vi "LoadCellTest.vi"() -> ()   [LabVIEW 2016]
uses:
  ModbusFactory/ModbusFactory.lvclass
  Common_RT_HPILC/HPILCFactory/HPILCFactory.lvclass
  Common_RT_HPILC/DataTypes/HPSettings.ctl
  Common_RT_ILC/DataTypes/ILCSettings.ctl
  Common_RT_ILC/DataTypes/ILCTimings.ctl
  Common_RT_HPILC/DataTypes/HPTimings.ctl
  ModbusFactory/ModbusFactory.lvclass/ModbusFactory.ctl
  Common_RT_ILC/ILC/ILC.lvclass/ILC.ctl
  <vilib>/Platform/TimedLoop/XDataNode/timing_clust.ctl
  <vilib>/Platform/TimedLoop/XDataNode/nitl_modes.ctl
  <vilib>/Platform/TimedLoop/XDataNode/wakeup.ctl
  Common_RT_Modbus/DynamicFrameParser/DynamicFrameParser.lvclass
  Common_RT_HPILC/HPILC/HPILC.lvclass/HPILC.ctl
  Common_RT_HPILC/HPILC/HPILC.lvclass
  D:/Code/Common_RT_ILC/ILC/ILC.lvclass
  <vilib>/FPGAPlugInAG/cRIO-9038/niLvFpga_Open_cRIO-9038.vi
  <vilib>/rvi/interface/common/dynamic/niFpgaDynamicAddResources.vi
  <vilib>/FPGAPlugInAG/Dynamic/niLvFpga_Abort_Dynamic.vi
  <vilib>/FPGAPlugInAG/Dynamic/niLvFpga_Reset_Dynamic.vi
  <vilib>/FPGAPlugInAG/Dynamic/niLvFpga_Run_Dynamic.vi
  <vilib>/Utility/error.llb/Error Cluster From Error Code.vi
  <vilib>/rvi/errors/niLvFpgaAdjustHostInterfaceError.vi
  <vilib>/FPGAPlugInAG/Dynamic/niLvFpga_Close_Dynamic.vi
  <vilib>/rvi/interface/nirviOpenFPGA/nirviOpenFPGA.xnode
  FPGA Bitfiles/modbus1Port.lvbitx
  FPGA/main.vi
  <vilib>/rvi/interface/nirviMethod/nirviMethod.xnode
  <vilib>/platform/TimedLoop/XDataNode/XDataNode.xnode
  <vilib>/rvi/interface/nirviCloseFPGA/nirviCloseFPGA.xnode
  Common_RT_Modbus/IModbus/IModbus.lvclass
  Common_RT_ILC/ILC/ILC.lvclass
  Common_RT_HPILC/RTHPILC.lvlib
  Common_RT_ILC/RTILC.lvlib
  <vilib>/FPGAPlugInAG/Dynamic/niLvFpga_ReadFifo_Dynamic.vi
  <vilib>/rvi/errors/niLvFpgaMergeErrorWithErrorCode.vi
  <vilib>/Platform/TimedLoop/XDataNode/XDNodeRunTimeDep.lvlib
panel:
  in  "Stop":bool
  out "Iteration":i32
  out "Array":sgl[](array[numeric])
  out "error out":errorcluster
  # "Port 1 = Modbus"
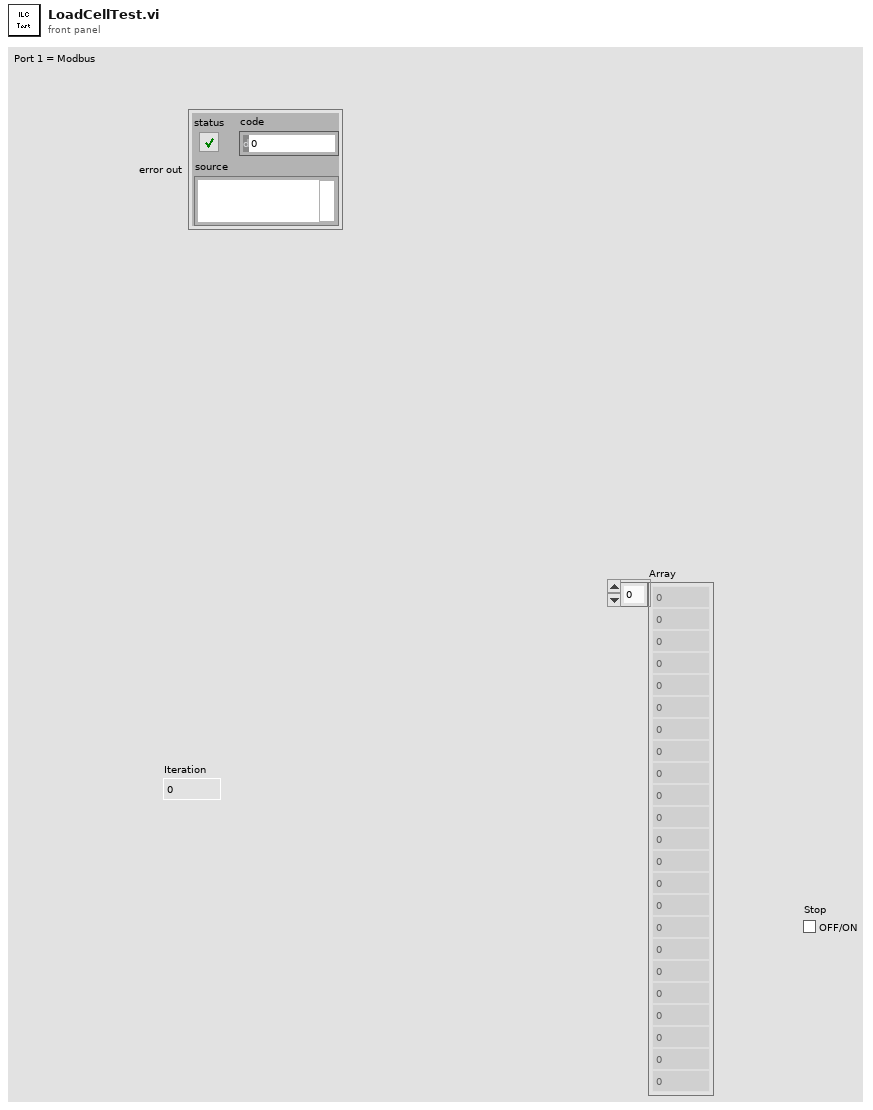
[diagram p1: front panel]
types:
  T1 = typedef "RTHPILC.lvlib/HPTimings.ctl" = cluster{"BroadcastStepMotor":u32, "ForceAndStatus":u32, "FreezeSensorValues":u32, "StepMotor":u32}
  T2 = typedef "RTILC.lvlib/ILCTimings.ctl" = cluster{"ADCOffsetSensitivity":u32, "ADCScanRate":u32, "ILCMode":u32, "ReadCalibration":u32, "ReportServerID":u32, "ReportServerStatus":u32, "Reset":u32, "SetTemporaryAddress":u32}
  T3 = typedef "RTHPILC.lvlib/HPSettings.ctl" = cluster{"ILCSettings":T4, "ID":i16, "ReferencePosition":i32}
  T4 = typedef "RTILC.lvlib/ILCSettings.ctl" = cluster{"Subnet":u8, "Address":u8}
  T5 = typedef "XDNodeRunTimeDep.lvlib/timing_clust.ctl" = cluster{"Expected End [f-1]":u64, "Actual End [f-1]":u64, "Finished Late? [f-1]":bool, "Expected End [i-1]":u64, "Actual End [i-1]":u64, "Finished Late? [i-1]":bool, "Expected Start [i]":u64, "Actual Start [i]":u64, "Expected Start [f]":u64, "Actual Start [f]":u64, "Source Name":string, "Structure Name":string, "Period":i64, "Deadline":i64, "Offset":i64, "Start":i64, "Priority":i32, "Timeout":i32, "Mode":T6, "Wakeup Reason":T7, "Error":errorcluster, "Source Type":string, "Secondary Source Type":string, "Global End Time":u64, "Global Start Time":u64, "Frame Duration":u64, "Iteration Duration":u64, "Assigned CPU":i32, "I/O Scan Engine Mode":u32}
  T6 = typedef "XDNodeRunTimeDep.lvlib/nitl_modes.ctl" = enum32{"No Change", "Process missed periods, maintain original phase", "Discard missed periods, maintain original phase", "Process missed periods, ignore original phase", "Discard missed periods, ignore original phase"}
  T7 = typedef "XDNodeRunTimeDep.lvlib/wakeup.ctl" = enum32{"Normal", "Aborted", "Asynchronous wakeup", "Timing source error", "Timed loop error", "Timeout"}
  T8 = typedef "RTILC.lvlib/ILCData.ctl" = cluster{"Constants":T9, "Command":T10, "Telemetry":T12, "Responses":T13, "Timings":T2}
  T9 = typedef "RTILC.lvlib/ILCConstants.ctl" = cluster{"Subnet":u8, "Address":u8}
  T10 = typedef "RTILC.lvlib/ILCCommand.ctl" = cluster{"ILCMode":u16, "TemporaryAddress":u8, "ADCScanRate":T11, "ADCChannel":u8, "ADCOffset":sgl, "ADCSensitivity":sgl}
  T11 = typedef "RTILC.lvlib/ILCScanRates.ctl" = u8
  T12 = typedef "RTILC.lvlib/ILCTelemetry.ctl" = cluster{"UniqueID":u64, "FirmwareType":u8, "NetworkNodeType":u8, "ILCOption":u8, "NetworkNodeOption":u8, "MajorRevision":u8, "MinorRevision":u8, "FirmwareName":string, "ILCMode":u16, "MajorFault":bool, "MinorFault":bool, "FaultOverride":bool, "UniqueIDCRCMismatch":bool, "AppTypeNodeTypeMismatch":bool, "AppMissing":bool, "AppCRCMismatch":bool, "TEDSNotFound":bool, "TEDS1Mismatch":bool, "TEDS2Mismatch":bool, "WatchdogResetDetected":bool, "BrownoutDetected":bool, "EventTrapResetDetected":bool, "TemporaryAddress":u8, "ADCScanRate":T11, "DAC1":u16, "DAC2":u16, "DAC3":u16, "DAC4":u16, "MainADCCalibrationK":sgl[], "MainSensorOffset":sgl[], "MainSensorSensitivity":sgl[], "BackupADCCalibrationK":sgl[], "BackupSensorOffset":sgl[], "BackupSensorSensitivity":sgl[]}
  T13 = typedef "RTILC.lvlib/ILCResponses.ctl" = cluster{"ReportServerID":T14, "ReportServerStatus":T14, "ILCMode":T14, "SetTemporaryAddress":T14, "Reset":T14, "ADCScanRate":T14, "ADCOffsetSensitivity":T14, "ReadDAC":T14, "ReadCalibration":T14}
  T14 = typedef "RTModbus.lvlib/ExceptionCodes.ctl" = u16
  T15 = typedef "RTModbus.lvlib/TxFrame.ctl" = cluster{"Data":u8[], "WaitForTrigger":bool, "WaitForRx":u16, "TriggerIRQ":bool, "DelayMicroseconds":u16, "DelayMilliseconds":u16, "Timestamp":bool}
  T16 = typedef "RTModbus.lvlib/RxFrame.ctl" = cluster{"Data":u8[], "Timestamp":u64}
  T17 = typedef "RTHPILC.lvlib/HPData.ctl" = cluster{"Constants":T18, "Command":T19, "Telemetry":T20, "Responses":T21, "Timings":T1}
  T18 = typedef "RTHPILC.lvlib/HPConstants.ctl" = cluster{"ID":i16, "ReferencePosition":i32}
  T19 = typedef "RTHPILC.lvlib/HPCommand.ctl" = cluster{"Steps":i8}
  T20 = typedef "RTHPILC.lvlib/HPTelemetry.ctl" = cluster{"ILCFault":bool, "LimitSwitchCWOperated":bool, "LimitSwitchCCWOperated":bool, "BroadcastCounter":u8, "SSIEncoderValue":i32, "LoadCellForce":sgl}
  T21 = typedef "RTHPILC.lvlib/HPResponses.ctl" = cluster{"StepMotor":T14, "ForceAndStatus":T14}
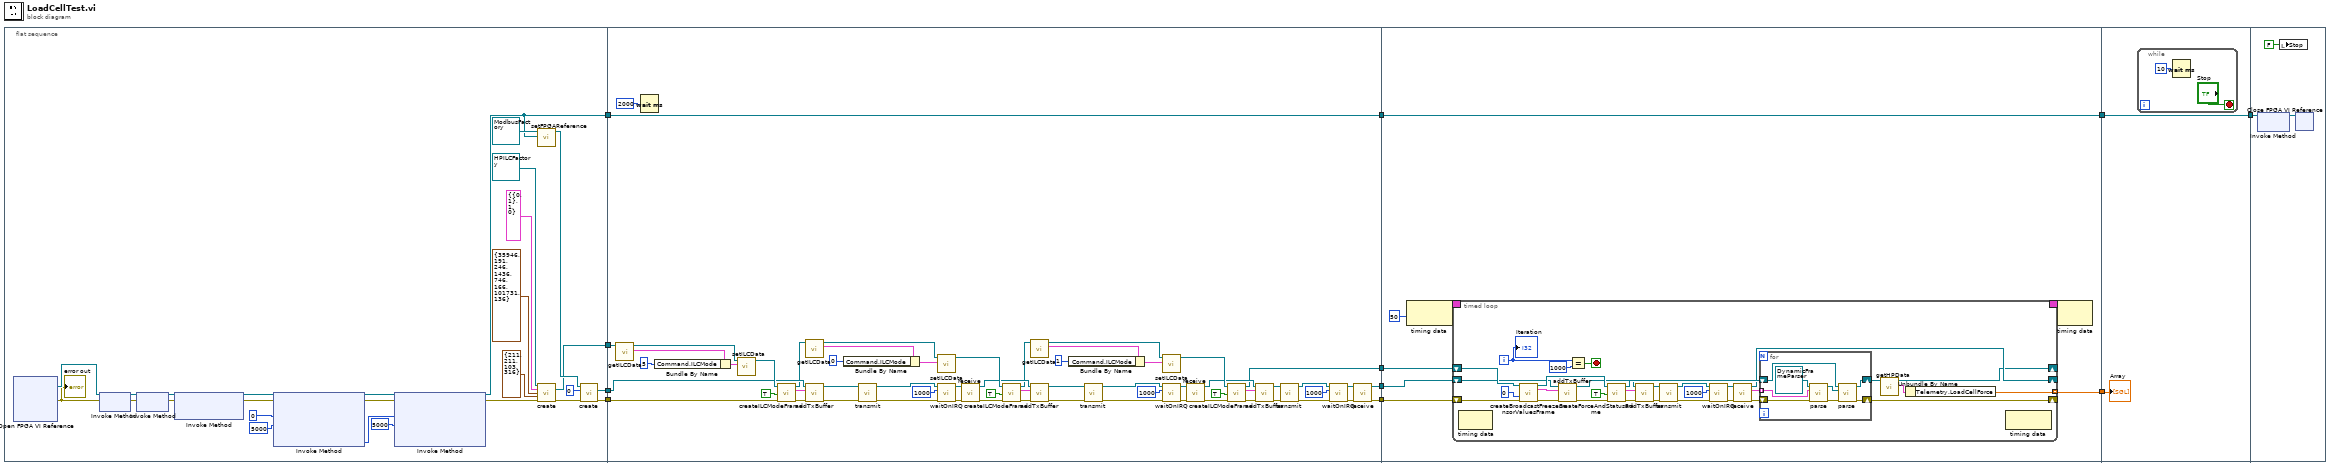
[diagram p0: block diagram]
diagram:
  n1 = flat-sequence {
    tunnel: [w15] -> w11
    tunnel: [w14] -> w10
    tunnel: [w13] -> w9
    tunnel: [w12] -> w7
    tunnel: w11 -> [w88]
    tunnel: w10 -> [w96]
    tunnel: w9 -> [w89]
    tunnel: [w42] -> w8
    tunnel: w7 -> [w42]
    tunnel: [w41] -> w6
    tunnel: [w40] -> w5
    tunnel: [w39] -> w4
    tunnel: [w105] -> w3
    tunnel: w8 -> [w105]
    tunnel: w6 -> [w101]
    tunnel: w5 -> [w99]
    tunnel: w4 -> [w100]
    tunnel: [w98] -> w1
    tunnel: w3 -> [w152]
    tunnel: [w152] -> w2
    tunnel: w1 -> [w151]
    tunnel: w2 -> [w156]
    frame #0 {
      n2 = xnode "Open FPGA VI Reference"() -> ("FPGA VI Reference Out"=w36:refnum<k20>, "error out"=w24:errorcluster)  [unwired: 2 in]
      "error out" <- w24
      n3 = xnode "Invoke Method"("FPGA VI Reference In"=w36, "error in"=w24) -> ("FPGA VI Reference Out"=w38:refnum<k20>, "error out"=w37:errorcluster)
      n4 = xnode "Invoke Method"("FPGA VI Reference In"=w38, "error in"=w37) -> ("FPGA VI Reference Out"=w28:refnum<k20>, "error out"=w26:errorcluster)
      n5 = xnode "Invoke Method"("FPGA VI Reference In"=w28, "error in"=w26) -> ("FPGA VI Reference Out"=w27:refnum<k20>, "error out"=w25:errorcluster)  [unwired: 1 in]
      n6 = xnode "Invoke Method"("FPGA VI Reference In"=w27, "error in"=w25, "Number of Elements"=u32 0, "Timeout (ms)"=5000) -> ("FPGA VI Reference Out"=w31:refnum<k20>, "error out"=w29:errorcluster, "Elements Remaining"=w32:u32)  [unwired: 1 out]
      n7 = xnode "Invoke Method"("FPGA VI Reference In"=w31, "error in"=w29, "Number of Elements"=w32, "Timeout (ms)"=5000) -> ("FPGA VI Reference Out"=w12:refnum<k20>, "error out"=w17:errorcluster)  [unwired: 2 out]
      n8 = call "setFPGAReference.vi"("FPGAReference"=w12, "ModbusFactory in"=refnum<class "ModbusFactory.lvclass"> refnum ("ModbusFactory.lvclass")) -> ("ModbusFactory out"=w19:refnum<class "ModbusFactory.lvclass">)  [unwired: 9 in]
      n9 = call "create.vi"("HardPointActuatorFactory in"=refnum<class "HPILCFactory.lvclass"> refnum ("RTHPILC.lvlib:HPILCFactory.lvclass"), "HPSettings"=T3 {"ILCSettings"={"Subnet"=0, "Address"=1}, "ID"=1, "ReferencePosition"=0}, "ILCTimings"=T2 {"ADCOffsetSensitivity"=35946, "ADCScanRate"=191, "ILCMode"=246, "ReadCalibration"=1436, "ReportServerID"=746, "ReportServerStatus"=166, "Reset"=101731, "SetTemporaryAddress"=136}, "HPTimings"=T1 {"BroadcastStepMotor"=211, "ForceAndStatus"=211, "FreezeSensorValues"=103, "StepMotor"=316}, "error in (no error)"=w17) -> ("HardPointActuator"=w14:refnum<class "HPILC.lvclass">, "error out"=w16:errorcluster)  [unwired: 8 in, 1 out]
      n10 = call-dynamic "create.vi"("error in (no error)"=w16, "Port"=0, "ModbusFactory in"=w19) -> ("error out"=w13:errorcluster, "Modbus"=w15:refnum<class "IModbus.lvclass">)  [unwired: 6 in, 1 out]
    }
    frame #1 {
      n11 = call "getILCData.vi"("ILC in"=w96) -> ("ILCData"=w95:T8, "ILC out"=w92:refnum<class "HPILC.lvclass">)  [unwired: 9 in]
      n12 = Wait (ms)(milliseconds to wait=u32 2000) -> ()  [unwired: 1 out]
      n13 = Bundle By Name(cluster=w95, "Command.ILCMode"=u16 5) -> (w93:T8)
      n14 = call "setILCData.vi"("ILCData"=w93, "ILC in"=w92) -> ("ILC out"=w91:refnum<class "HPILC.lvclass">)  [unwired: 9 in]
      n15 = call "createILCModeFrame.vi"("error in (no error)"=w89, "TriggerIRQ"=TRUE, "ILC in"=w91) -> ("error out"=w86:errorcluster, "Frame"=w87:T15, "ILC out"=w64:refnum<class "HPILC.lvclass">)  [unwired: 6 in]
      n16 = call "getILCData.vi"("ILC in"=w64) -> ("ILCData"=w65:T8, "ILC out"=w67:refnum<class "HPILC.lvclass">)  [unwired: 9 in]
      n17 = call-dynamic "addTxBuffer.vi"("error in (no error)"=w86, "TxFrame"=w87, "IModbus in"=w88) -> ("error out"=w82:errorcluster, "IModbus out"=w85:refnum<class "IModbus.lvclass">)  [unwired: 7 in]
      n18 = Bundle By Name(cluster=w65, "Command.ILCMode"=u16 0) -> (w61:T8)
      n19 = call-dynamic "transmit.vi"("error in (no error)"=w82, "IModbus in"=w85) -> ("error out"=w81:errorcluster, "IModbus out"=w84:refnum<class "IModbus.lvclass">)  [unwired: 8 in]
      n20 = call "setILCData.vi"("ILCData"=w61, "ILC in"=w67) -> ("ILC out"=w68:refnum<class "HPILC.lvclass">)  [unwired: 9 in]
      n21 = call-dynamic "waitOnIRQ.vi"("error in (no error)"=w81, "Timeout"=1000, "IModbus in"=w84) -> ("error out"=w79:errorcluster, "IModbus out"=w83:refnum<class "IModbus.lvclass">)  [unwired: 5 in, 2 out]
      n22 = call-dynamic "receive.vi"("error in (no error)"=w79, "IModbus in"=w83) -> ("error out"=w62:errorcluster, "IModbus out"=w63:refnum<class "IModbus.lvclass">)  [unwired: 7 in, 1 out]
      n23 = call "createILCModeFrame.vi"("error in (no error)"=w62, "TriggerIRQ"=TRUE, "ILC in"=w68) -> ("error out"=w71:errorcluster, "Frame"=w70:T15, "ILC out"=w44:refnum<class "HPILC.lvclass">)  [unwired: 6 in]
      n24 = call "getILCData.vi"("ILC in"=w44) -> ("ILCData"=w59:T8, "ILC out"=w57:refnum<class "HPILC.lvclass">)  [unwired: 9 in]
      n25 = call-dynamic "addTxBuffer.vi"("error in (no error)"=w71, "TxFrame"=w70, "IModbus in"=w63) -> ("error out"=w75:errorcluster, "IModbus out"=w72:refnum<class "IModbus.lvclass">)  [unwired: 7 in]
      n26 = Bundle By Name(cluster=w59, "Command.ILCMode"=u16 1) -> (w60:T8)
      n27 = call-dynamic "transmit.vi"("error in (no error)"=w75, "IModbus in"=w72) -> ("error out"=w76:errorcluster, "IModbus out"=w73:refnum<class "IModbus.lvclass">)  [unwired: 8 in]
      n28 = call "setILCData.vi"("ILCData"=w60, "ILC in"=w57) -> ("ILC out"=w56:refnum<class "HPILC.lvclass">)  [unwired: 9 in]
      n29 = call-dynamic "waitOnIRQ.vi"("error in (no error)"=w76, "Timeout"=1000, "IModbus in"=w73) -> ("error out"=w78:errorcluster, "IModbus out"=w74:refnum<class "IModbus.lvclass">)  [unwired: 5 in, 2 out]
      n30 = call-dynamic "receive.vi"("error in (no error)"=w78, "IModbus in"=w74) -> ("error out"=w43:errorcluster, "IModbus out"=w45:refnum<class "IModbus.lvclass">)  [unwired: 7 in, 1 out]
      n31 = call "createILCModeFrame.vi"("error in (no error)"=w43, "TriggerIRQ"=TRUE, "ILC in"=w56) -> ("error out"=w53:errorcluster, "Frame"=w54:T15, "ILC out"=w40:refnum<class "HPILC.lvclass">)  [unwired: 6 in]
      n32 = call-dynamic "addTxBuffer.vi"("error in (no error)"=w53, "TxFrame"=w54, "IModbus in"=w45) -> ("error out"=w49:errorcluster, "IModbus out"=w52:refnum<class "IModbus.lvclass">)  [unwired: 7 in]
      n33 = call-dynamic "transmit.vi"("error in (no error)"=w49, "IModbus in"=w52) -> ("error out"=w48:errorcluster, "IModbus out"=w51:refnum<class "IModbus.lvclass">)  [unwired: 8 in]
      n34 = call-dynamic "waitOnIRQ.vi"("error in (no error)"=w48, "Timeout"=1000, "IModbus in"=w51) -> ("error out"=w46:errorcluster, "IModbus out"=w50:refnum<class "IModbus.lvclass">)  [unwired: 5 in, 2 out]
      n35 = call-dynamic "receive.vi"("error in (no error)"=w46, "IModbus in"=w50) -> ("error out"=w41:errorcluster, "IModbus out"=w39:refnum<class "IModbus.lvclass">)  [unwired: 7 in, 1 out]
    }
    frame #2 {
      n36 = node-c288(i64 50 ("Period")) -> (w104:T5)
      n37 = timed-loop {
        timing: w104 -> [_]
        timing-out: [_] -> w103
        shift-right: [w106] -> _
        shift-left: w101 -> [w131]
        shift-right: [w111] -> _
        shift-left: w100 -> [w116]
        shift-right: [w107] -> _
        shift-left: w99 -> [w133]
        tunnel: [w108] -> w98 mode=indexing
        i -> [w136]
        stop <- w134 stop-if-true
        n38 = node-c288() -> ()  [unwired: 1 in, 1 out]
        n39 = call "createBroadcastFreezeSensorValuesFrame.vi"("HardPointActuator in"=w133, "BroadcastCounter"=u8 0, "error in (no error)"=w131) -> ("HardPointActuator out"=w121:refnum<class "HPILC.lvclass">, "Frame"=w130:T15, "error out"=w129:errorcluster)  [unwired: 10 in]
        n40 = call-dynamic "addTxBuffer.vi"("error in (no error)"=w129, "TxFrame"=w130, "IModbus in"=w116) -> ("error out"=w128:errorcluster, "IModbus out"=w117:refnum<class "IModbus.lvclass">)  [unwired: 7 in]
        n41 = Equal?(x=w136, y=1000) -> (x = y?=w134:bool)
        n42 = call "createForceAndStatusFrame.vi"("error in (no error)"=w128, "TriggerIRQ"=TRUE, "HardPointActuator in"=w121) -> ("error out"=w127:errorcluster, "Frame"=w126:T15, "HardPointActuator out"=w118:refnum<class "HPILC.lvclass">)  [unwired: 6 in]
        n43 = call-dynamic "addTxBuffer.vi"("error in (no error)"=w127, "TxFrame"=w126, "IModbus in"=w117) -> ("error out"=w125:errorcluster, "IModbus out"=w115:refnum<class "IModbus.lvclass">)  [unwired: 7 in]
        n44 = call-dynamic "transmit.vi"("error in (no error)"=w125, "IModbus in"=w115) -> ("error out"=w124:errorcluster, "IModbus out"=w114:refnum<class "IModbus.lvclass">)  [unwired: 8 in]
        n45 = call-dynamic "waitOnIRQ.vi"("error in (no error)"=w124, "Timeout"=1000, "IModbus in"=w114) -> ("error out"=w123:errorcluster, "IModbus out"=w112:refnum<class "IModbus.lvclass">)  [unwired: 5 in, 2 out]
        n46 = call-dynamic "receive.vi"("error in (no error)"=w123, "IModbus in"=w112) -> ("error out"=w119:errorcluster, "Data"=w120:T16[], "IModbus out"=w111:refnum<class "IModbus.lvclass">)  [unwired: 7 in]
        n47 = for {
          tunnel: w120 -> [w143] mode=indexing
          shift-right: [w137] -> w106
          shift-left: w119 -> [w142]
          shift-right: [w138] -> w110
          shift-left: w118 -> [w139]
          n48 = call "parse.vi"("error in (no error)"=w142, "RxFrame"=w143, "FrameParser in"=refnum<class "DynamicFrameParser.lvclass"> refnum ("RTModbus.lvlib:DynamicFrameParser.lvclass")) -> ("error out"=w141:errorcluster, "FrameParser out"=w140:refnum<class "DynamicFrameParser.lvclass">)  [unwired: 7 in]
          n49 = call-dynamic "parse.vi"("error in (no error)"=w141, "DynamicFrameParser"=w140, "HPILC in"=w139) -> ("error out"=w137:errorcluster, "HPILC out"=w138:refnum<class "HPILC.lvclass">)  [unwired: 6 in, 1 out]
        }
        n50 = call "getHPData.vi"("HardPointActuator in"=w110) -> ("HPData"=w109:T17, "HardPointActuator out"=w107:refnum<class "HPILC.lvclass">)  [unwired: 9 in]
        n51 = Unbundle By Name(w109) -> ("Telemetry.LoadCellForce"=w108:sgl)
        n52 = node-c288() -> ()  [unwired: 1 in, 1 out]
        "Iteration" <- w136
      }
      n53 = node-c288(w103) -> ()  [unwired: 1 out]
    }
    frame #3 {
      n54 = while {
        stop <- "Stop" stop-if-true
        n55 = Wait (ms)(milliseconds to wait=u32 10) -> ()  [unwired: 1 out]
      }
      "Array" <- w151
    }
    frame #4 {
      n56 = xnode "Invoke Method"("FPGA VI Reference In"=w156) -> ("FPGA VI Reference Out"=w157:refnum<k20>)  [unwired: 1 in, 1 out]
      n57 = local write "Stop"(FALSE ("Stop")) -> ()
      n58 = xnode "Close FPGA VI Reference"("FPGA VI Reference In"=w157) -> ()  [unwired: 1 in, 1 out]
    }
  }
